vi "Math channels.vi"(6 "dt":dbl=1.0 format="%0.2f", 8 "b":dbl, 9 "a":dbl, 10 "Magnitude":dbl[][](array[numeric]), 11 "Phase":dbl[][](array[numeric])) -> (2 "Magnitude +Math":dbl[][](array[numeric]), 3 "Phase + Math":dbl[][](array[numeric]))   [LabVIEW 2013]
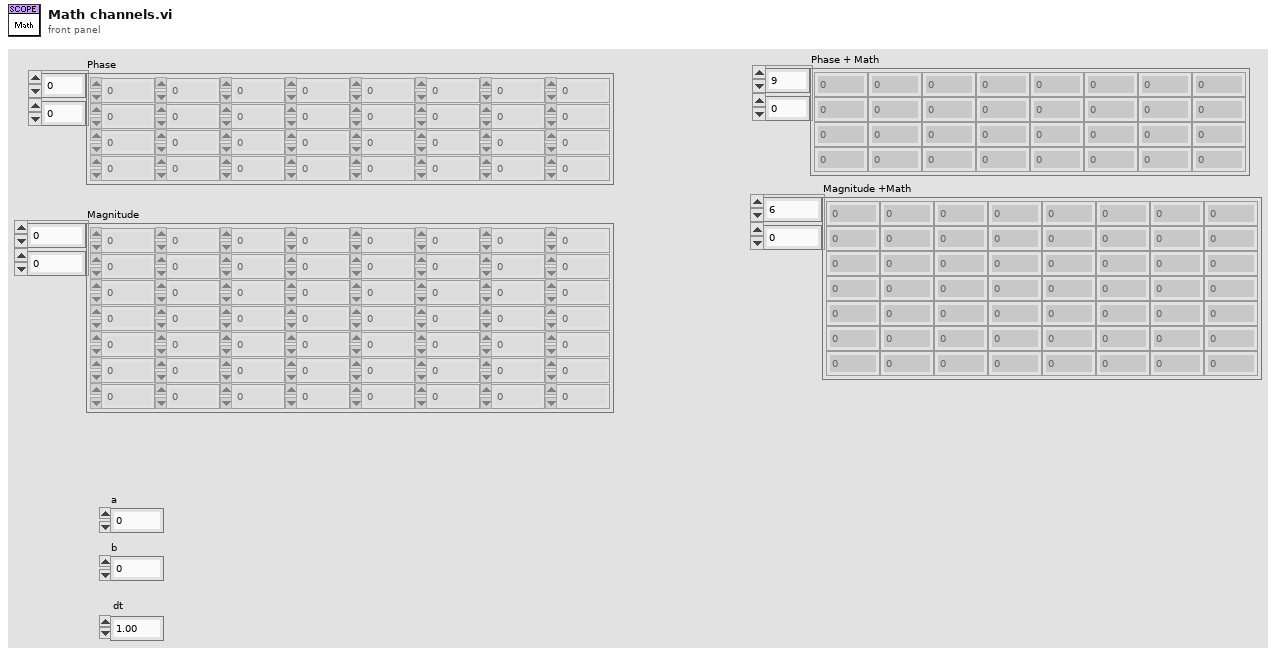
[diagram p1: front panel]
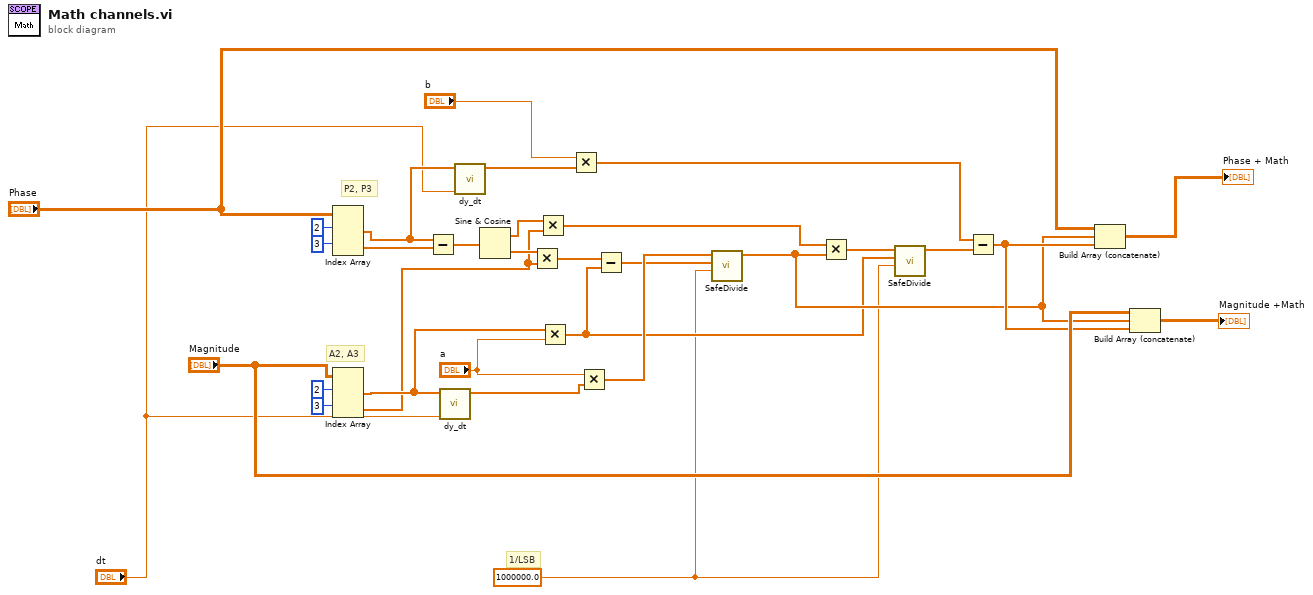
[diagram p0: block diagram]
diagram:
  w1 = 1000000.0
  # "1/LSB"
  # "A2, A3"
  # "P2, P3"
  n1 = Index Array(array="Phase", index (row) #1=2 ("index (row)"), index (row) #2=3 ("index (row)")) -> (element #1=w20:dbl[], element #2=w26:dbl[])  [unwired: 2 in]
  n2 = Index Array(array="Magnitude", index (row) #1=2 ("index (row)"), index (row) #2=3 ("index (row)")) -> (element #1=w22:dbl[], element #2=w19:dbl[])  [unwired: 2 in]
  n3 = Subtract(x=w20, y=w26) -> (x-y=w25:dbl[])
  n4 = call "dy_dt.vi"("dt"="dt", "y"=w22) -> ("dy/dt"=w27:dbl[])  [unwired: 9 in]
  n5 = call "dy_dt.vi"("dt"="dt", "y"=w20) -> ("dy/dt"=w16:dbl[])  [unwired: 9 in]
  n6 = Sine & Cosine(0:w25) -> (1:w18:dbl[], 2:w24:dbl[])
  n7 = Multiply(x=w24, y=w19) -> (x*y=w23:dbl[])
  n8 = Multiply(x=w18, y=w19) -> (x*y=w17:dbl[])
  n9 = Multiply(x=w22, y="a") -> (x*y=w2:dbl[])
  n10 = Multiply(x="b", y=w16) -> (x*y=w14:dbl[])
  n11 = Multiply(x="a", y=w27) -> (x*y=w7:dbl[])
  n12 = Subtract(x=w23, y=w2) -> (x-y=w6:dbl[])
  n13 = call "SafeDivide.vi"("Max"=w1, "y"=w6, "x"=w7) -> ("x/y"=w5:dbl[])  [unwired: 8 in]
  n14 = Multiply(x=w17, y=w5) -> (x*y=w3:dbl[])
  n15 = call "SafeDivide.vi"("Max"=w1, "y"=w2, "x"=w3) -> ("x/y"=w4:dbl[])  [unwired: 8 in]
  n16 = Subtract(x=w14, y=w4) -> (x-y=w11:dbl[])
  n17 = Build Array (concatenate)("Phase", w5, w11) -> (→"Phase + Math":dbl[][])
  n18 = Build Array (concatenate)("Magnitude", w5, w11) -> (→"Magnitude +Math":dbl[][])
